vi "niWLAN - OPPO - 80211abgnIQMeasurements.vi"(0 "niwlan analysis session":T5, 2 "Measurement Type":T3(ring), 3 "PL":T2, 7 "TV Parameters(DataType)":T4 {"Standard" items=["80211A/G/J/P OFDM", "80211B/G DSSS", "80211G DSSSOFDM", "80211N MIMOOFDM", "80211AC MIMOOFDM"]; "OFDM Data Rate (Mbps)" items=["6", "9", "12", "18", "24", "36", "48", "54"]; "80211n PLCP Frame Format" items=["Mixed Format", "Greenfield Format"]; "FEC Coding Type" items=["BCC", "LDPC"]; "DSSS Data Rate (Mbps)" items=["1", "2", "5.5 CCK", "5.5 PBCC", "11 CCK", "11 PBCC", "22", "33"]}, 11 "error out":errorcluster) -> (4 "niWLAN session":T5, 6 "Spectrum Result":cluster{"SMM":dbl, "SMM VECTOR":dbl[]}, 8 "Mod Result":T1={"EVM"=-53.23630011850784, "RMS POWER"=-20.854257366141734, "FREQ ERR PPm"=0.0031004693085368165, "Clock ERR PPm"=1.9815491854025864}, 15 "error out":errorcluster)   [LabVIEW 2012]
uses:
  <vilib>/RF Toolkits/WLAN/analysis/controls/wlanv1 Analysis Refnum.ctl
  TV/RW/Includes/WLAN - TV - RW - INC - TV_DataType_Cluster.ctl
  TV/RW/Includes/WLAN - TV - RW - INC - Tx_IQModResult.ctl
  <resource>/objmgr/niWLANAnalysis.rc
panel:
  out "Waveform Graph":cluster{"f0":dbl, "df":dbl, "Y":dbl[]}[](graph)
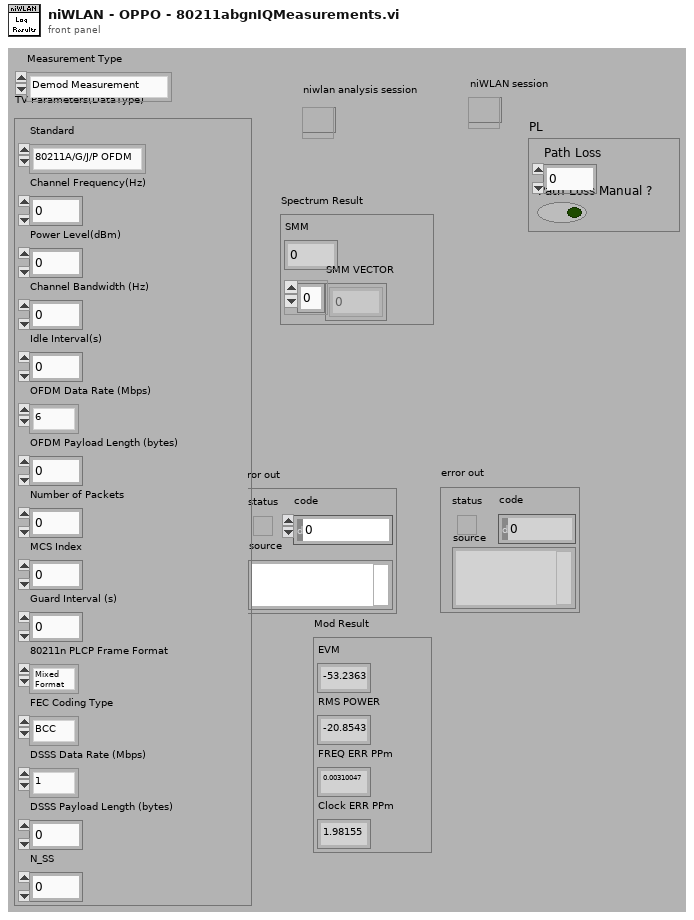
[diagram p1: front panel]
types:
  T1 = typedef "WLAN - TV - RW - INC - Tx_IQModResult.ctl" = cluster{"EVM":dbl, "RMS POWER":dbl, "FREQ ERR PPm":dbl, "Clock ERR PPm":dbl}
  T2 = cluster{"Path Loss":dbl, "Path Loss Manual ?":bool}
  T3 = enum16{"Demod Measurement", "Spectrum Measurement"}
  T4 = typedef "WLAN - TV - RW - INC - TV_DataType_Cluster.ctl" = cluster{"Standard":i32, "Channel Frequency(Hz)":dbl, "Power Level(dBm)":dbl, "Channel Bandwidth (Hz)":dbl, "Idle Interval(s)":dbl, "OFDM Data Rate (Mbps)":i32, "OFDM Payload Length (bytes)":i32, "Number of Packets":i32, "MCS Index":i32, "Guard Interval (s)":dbl, "80211n PLCP Frame Format":i32, "FEC Coding Type":i32, "DSSS Data Rate (Mbps)":i32, "DSSS Payload Length (bytes)":i32, "N_SS":i32}
  T5 = typedef "wlanv1 Analysis Refnum.ctl" = refnum<k20>
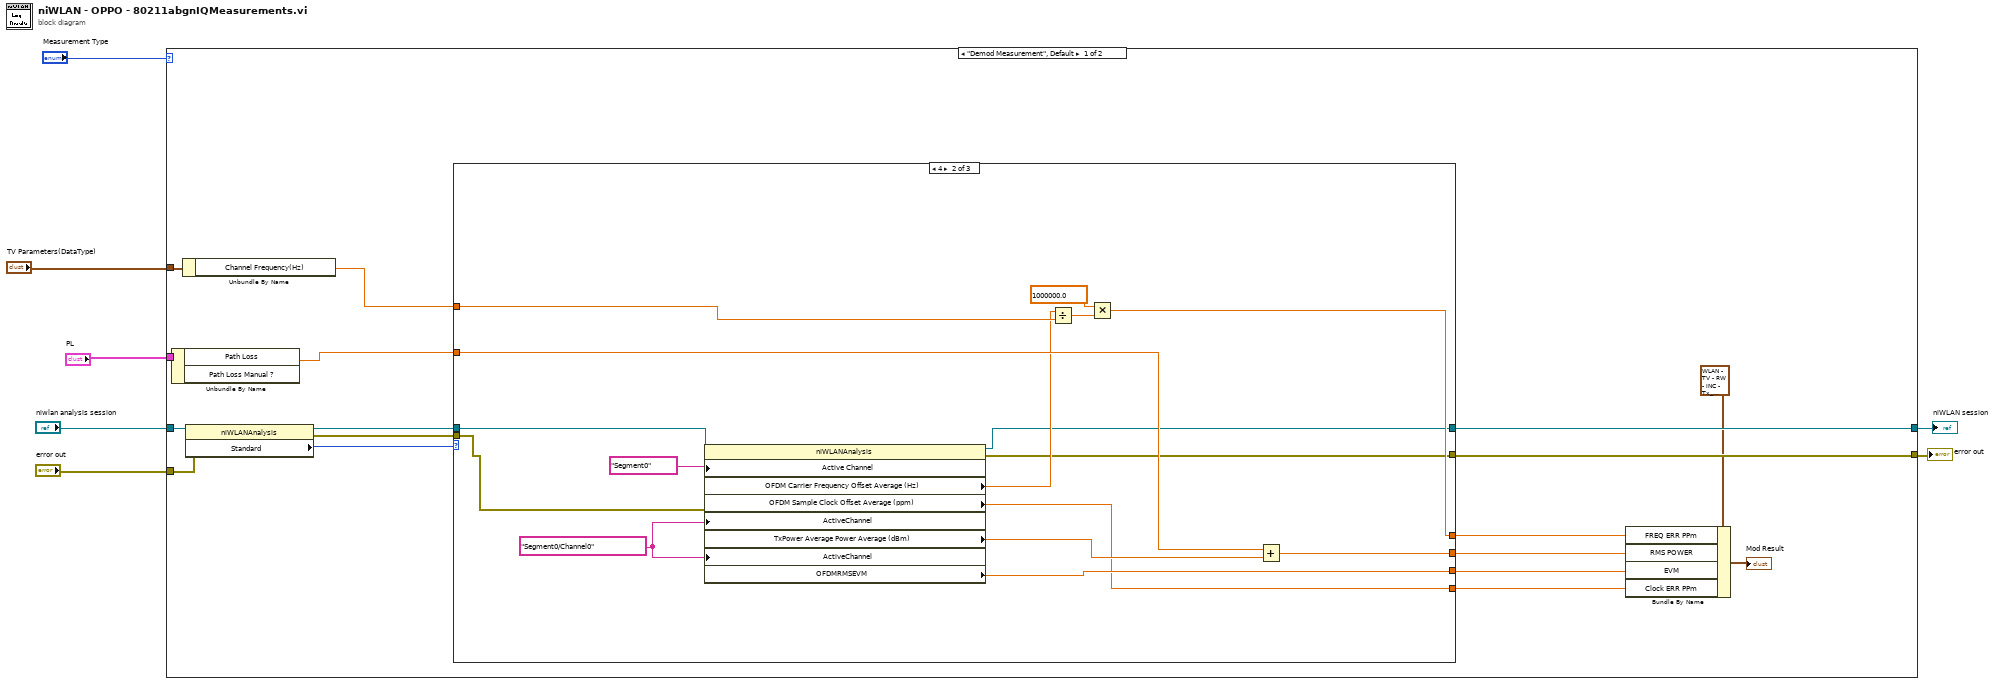
[diagram p0: block diagram]
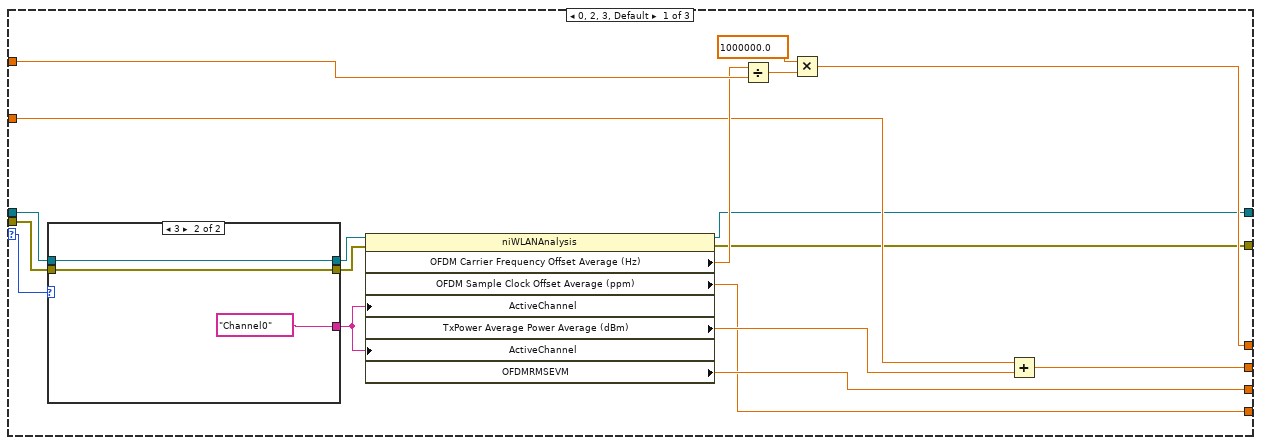
[diagram p2: hidden frame]
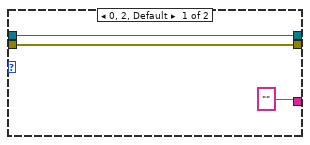
[diagram p3: hidden frame]
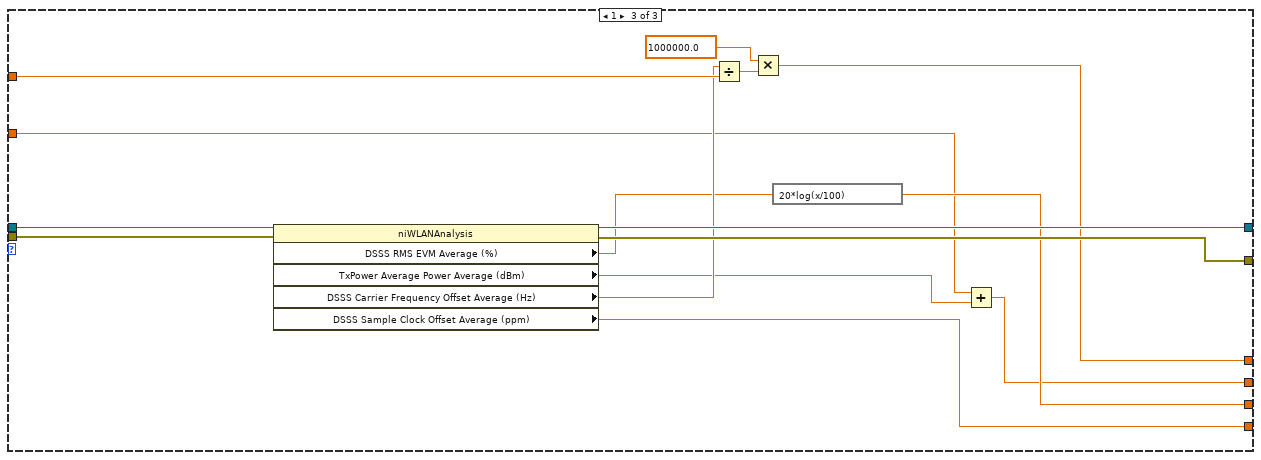
[diagram p4: hidden frame]
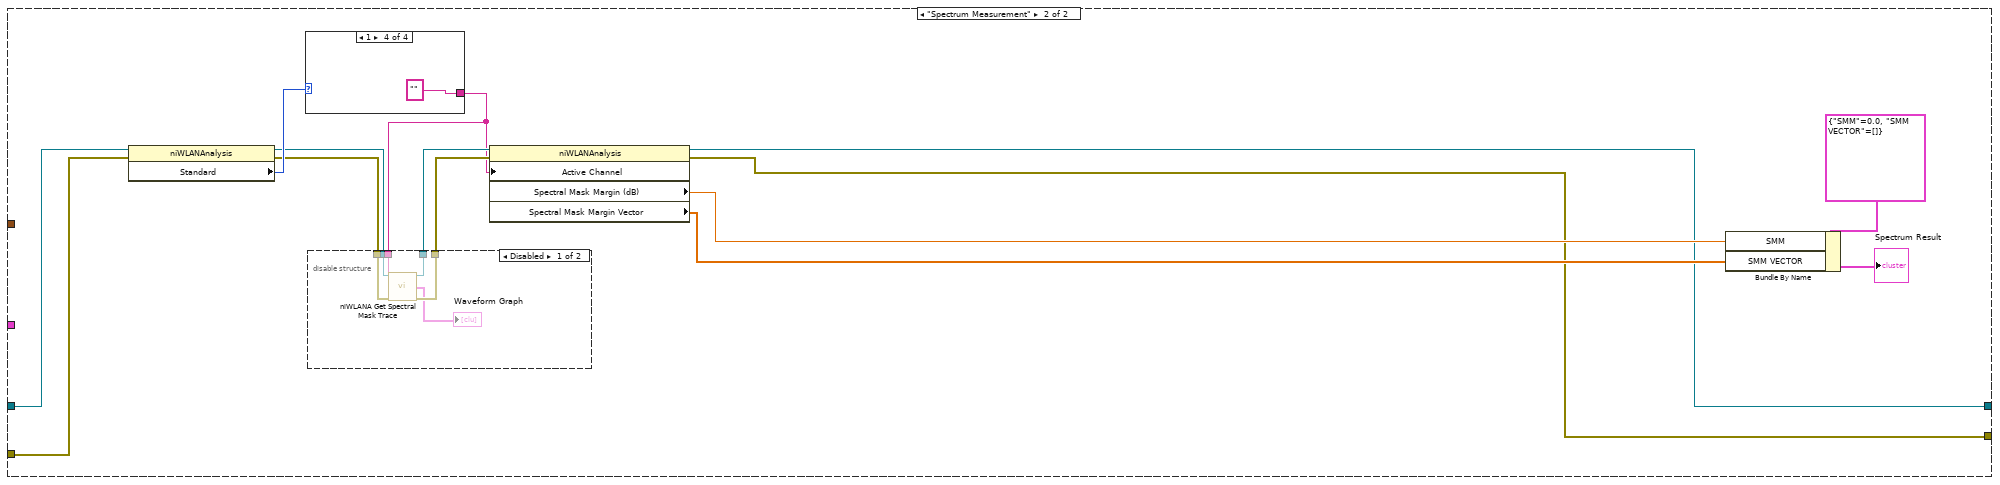
[diagram p5: hidden frame]
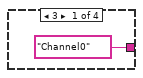
[diagram p7: hidden frame]
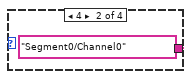
[diagram p8: hidden frame]
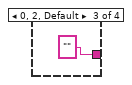
[diagram p9: hidden frame]
diagram:
  n1 = case shown="\"Demod Measurement\", Default" "Measurement Type" {
    tunnel: "niwlan analysis session" -> [w24 w92]
    tunnel: "error out" -> [w22 w93]
    tunnel: "TV Parameters(DataType)" -> [w20 _]
    tunnel: [w18 w86] -> w4
    tunnel: [w17 w85] -> w3
    tunnel: "PL" -> [w16 _]
    frame "Demod Measurement", Default {
      n2 = Unbundle By Name(w16) -> ("Path Loss"=w8:dbl)  [unwired: 1 out]
      n3 = Unbundle By Name(w20) -> ("Channel Frequency(Hz)"=w9:dbl)
      n4 = property class="niWLANAnalysis"(reference=w24, error in=w22) -> (reference out=w23:T5, error out=w21:errorcluster, "Standard"=w19:i32)
      n5 = case shown="4" w19 {
        selector: w19 -> [w42 _ _]
        tunnel: w21 -> [w38 w56 w78]
        tunnel: w23 -> [w30 w57 w79]
        tunnel: [w27 w52 w77] -> w18
        tunnel: [w26 w51 w76] -> w17
        tunnel: w9 -> [w39 w62 w75]
        tunnel: w8 -> [w34 w60 w68]
        tunnel: [w32 w58 w69] -> w14
        tunnel: [w35 w61 w70] -> w12
        tunnel: [w25 w49 w65] -> w15
        tunnel: [w33 w59 w67] -> w13
        frame 0, 2, 3, Default {
          n6 = case shown="3" w42 {
            tunnel: ["" ("Active Channel") "Channel0" ("Active Channel")] -> w37
            tunnel: w30 -> [w44 w46]
            tunnel: w38 -> [w43 w47]
            tunnel: [w43 w47] -> w31
            tunnel: [w44 w46] -> w29
            frame 0, 2, Default {
            }
            frame 3 {
            }
          }
          n7 = property class="niWLANAnalysis"(reference=w29, error in=w31, "ActiveChannel"=w37, "ActiveChannel"=w37) -> (reference out=w27:T5, error out=w26:errorcluster, "OFDM Carrier Frequency Offset Average (Hz)"=w36:dbl, "OFDM Sample Clock Offset Average (ppm)"=w25:dbl, "TxPower Average Power Average (dBm)"=w28:dbl, "OFDMRMSEVM"=w35:dbl)
          n8 = Divide(x=w36, y=w39) -> (x/y=w41:dbl)
          n9 = Multiply(x=1000000.0, y=w41) -> (x*y=w32:dbl)
          n10 = Add(x=w34, y=w28) -> (x+y=w33:dbl)
        }
        frame 4 {
          w53 = "Segment0/Channel0" ("Active Channel")
          n11 = property class="niWLANAnalysis"(reference=w57, error in=w56, "Active Channel"="Segment0", "ActiveChannel"=w53, "ActiveChannel"=w53) -> (reference out=w52:T5, error out=w51:errorcluster, "OFDM Carrier Frequency Offset Average (Hz)"=w55:dbl, "OFDM Sample Clock Offset Average (ppm)"=w49:dbl, "TxPower Average Power Average (dBm)"=w50:dbl, "OFDMRMSEVM"=w61:dbl)
          n12 = Divide(x=w55, y=w62) -> (x/y=w64:dbl)
          n13 = Multiply(x=1000000.0, y=w64) -> (x*y=w58:dbl)
          n14 = Add(x=w60, y=w50) -> (x+y=w59:dbl)
        }
        frame 1 {
          n15 = property class="niWLANAnalysis"(reference=w79, error in=w78) -> (reference out=w77:T5, error out=w76:errorcluster, "DSSS RMS EVM Average (%)"=w71:dbl, "TxPower Average Power Average (dBm)"=w66:dbl, "DSSS Carrier Frequency Offset Average (Hz)"=w72:dbl, "DSSS Sample Clock Offset Average (ppm)"=w65:dbl)
          n16 = Divide(x=w72, y=w75) -> (x/y=w74:dbl)
          n17 = Multiply(x=1000000.0, y=w74) -> (x*y=w69:dbl)
          n18 = expression code="20*log(x/100)"(w71) -> (w70:dbl)
          n19 = Add(x=w68, y=w66) -> (x+y=w67:dbl)
        }
      }
      n20 = Bundle By Name(cluster=T1 {"EVM"=-53.23630011850784, "RMS POWER"=-20.854257366141734, "FREQ ERR PPm"=0.0031004693085368165, "Clock ERR PPm"=1.9815491854025864} ("Mod Result"), "FREQ ERR PPm"=w14, "RMS POWER"=w13, "EVM"=w12, "Clock ERR PPm"=w15) -> (→"Mod Result":T1)
    }
    frame "Spectrum Measurement" {
      n21 = property class="niWLANAnalysis"(reference=w92, error in=w93) -> (reference out=w84:T5, error out=w83:errorcluster, "Standard"=w91:i32)
      n22 = case shown="1" w91 {
        tunnel: ["Channel0" ("active channel") "Segment0/Channel0" ("active channel") "" ("active channel") "" ("active channel")] -> w80
        frame 3 {
        }
        frame 4 {
        }
        frame 0, 2, Default {
        }
        frame 1 {
        }
      }
      n23 = disable-structure shown="Disabled" {
        disable-tunnel: w84 -> [w99 w101]
        disable-tunnel: w83 -> [w98 w100]
        disable-tunnel: [w97 w101] -> w82
        disable-tunnel: [w96 w100] -> w81
        disable-tunnel: w80 -> [w94 _]
        frame Disabled {
          n24 = call <vilib>:"niWLANA Get Spectral Mask Trace.vi"("niwlan analysis session"=w99, "active channel"=w94, "error in"=w98) -> ("niwlan analysis session out"=w97:T5, "spectral mask"=→"Waveform Graph":cluster{"f0":dbl, "df":dbl, "Y":dbl[]}[], "error out"=w96:errorcluster)  [unwired: 1 in, 9 out]
        }
        frame Enabled {
        }
      }
      n25 = property class="niWLANAnalysis"(reference=w82, error in=w81, "Active Channel"=w80) -> (reference out=w86:T5, error out=w85:errorcluster, "Spectral Mask Margin (dB)"=w89:dbl, "Spectral Mask Margin Vector"=w88:dbl[])
      n26 = Bundle By Name(cluster=cluster{"SMM":dbl, "SMM VECTOR":dbl[]} {"SMM"=0.0, "SMM VECTOR"=[]}, "SMM"=w89, "SMM VECTOR"=w88) -> (→"Spectrum Result":cluster{"SMM":dbl, "SMM VECTOR":dbl[]})
    }
  }
  "error out" <- w3
  "niWLAN session" <- w4
